vi "PFD_Heading.vi"(8 "Refresh Rate (Hz)":u32=30) -> ()   [LabVIEW 2023]
uses:
  <vilib>/Utility/miscctls.llb/LVBoundsTypeDef.ctl
  pfd_global.vi
panel:
  out "HDG":bool
  out "PFD_HeadingControl":sgl format="%#_13g"
  out "PFD_HeadingTop":picture
  out "PFD_Heading":picture
  out "PFD_HeadingBack":picture
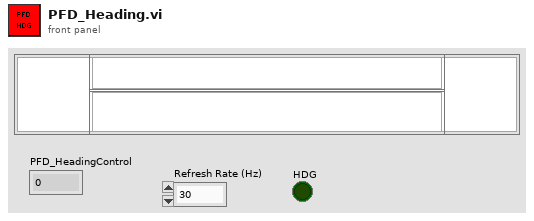
[diagram p1: front panel]
types:
  T1 = cluster{"left":i16, "top":i16, "right":i16, "bottom":i16}
  T2 = typedef "LVBoundsTypeDef.ctl" = cluster{"Width":u32, "Height":u32}
  T3 = cluster{"Font Name:":string, "Size":i16, "Strikeout?":bool, "Italic?":bool, "Underline?":bool, "Outline?":bool, "Shadow?":bool, "Bold?":bool}
  T4 = enum16{"User-specified Font", "Application Font", "System Font", "Dialog Font"}
  T5 = cluster{"horizontal":enum16{"left", "center", "right"}, "vertical":enum16{"top", "center", "bottom"}}
  T6 = cluster{cluster{i16, "x":i16}, cluster{i16, "x":i16}}
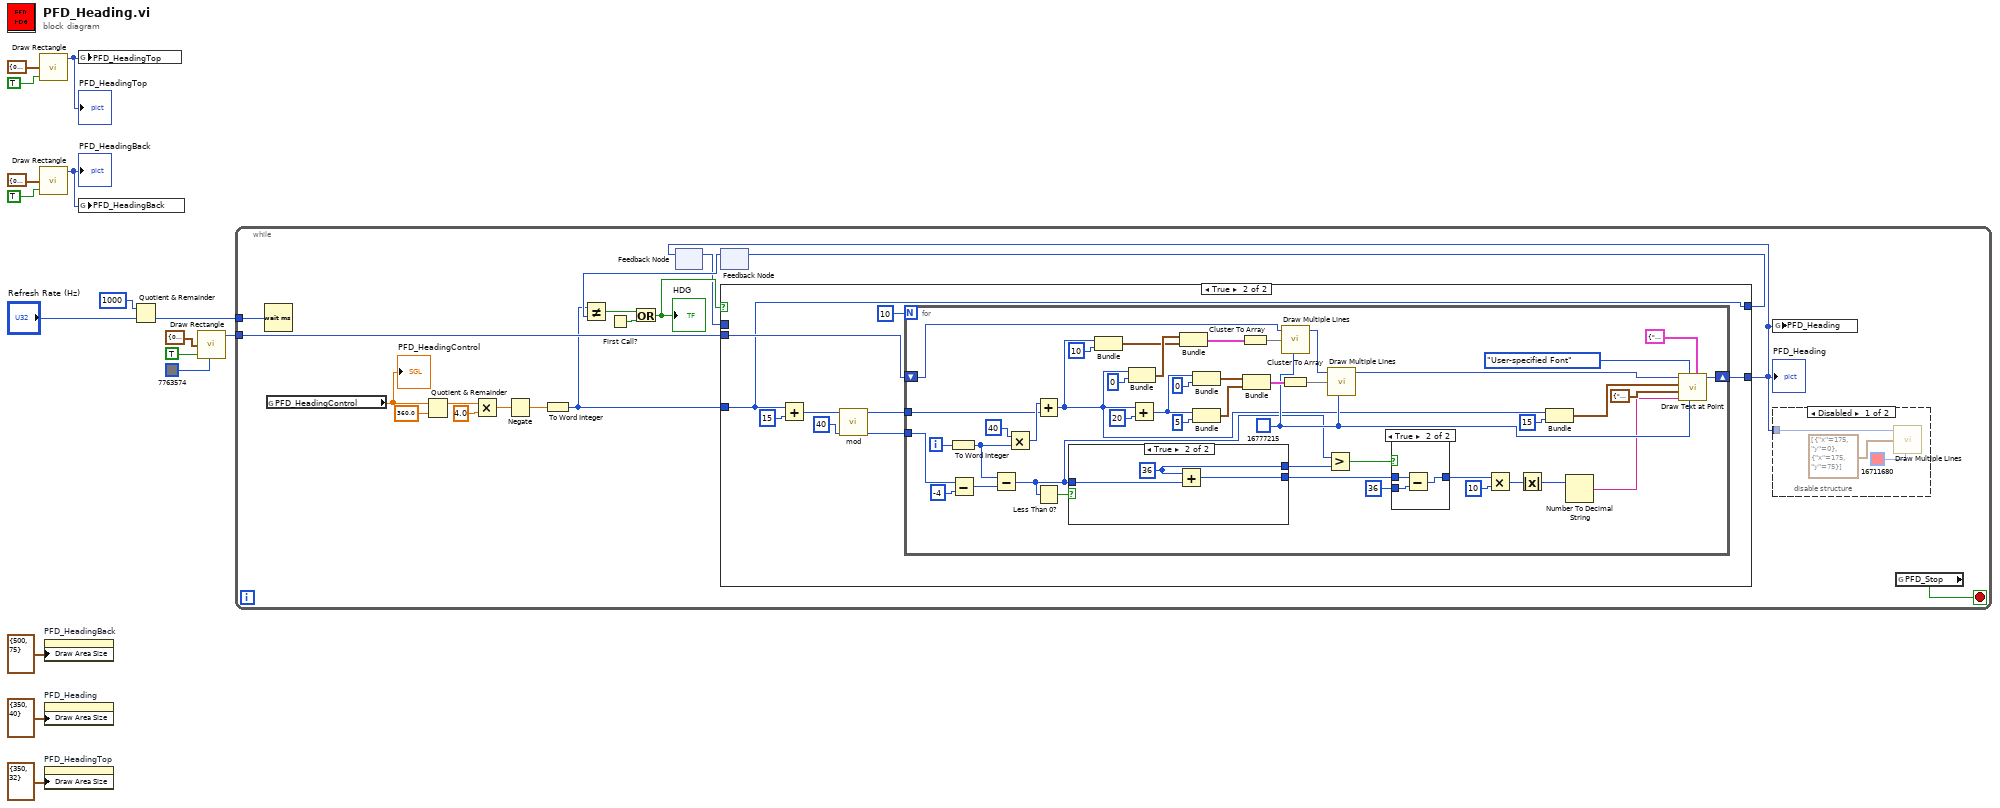
[diagram p0: block diagram]
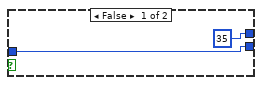
[diagram p5: hidden frame]
diagram:
  n1 = call <vilib>:"Draw Rectangle.vi"("rect"=T1 {"left"=0, "top"=0, "right"=350, "bottom"=52}, "fill?(F)"=TRUE) -> ("new picture"=w2:picture)  [unwired: 7 in]
  "PFD_HeadingTop" <- w2
  n2 = call <vilib>:"Draw Rectangle.vi"("rect"=T1 {"left"=0, "top"=0, "right"=500, "bottom"=75}, "fill?(F)"=TRUE) -> ("new picture"=w1:picture)  [unwired: 7 in]
  "PFD_HeadingBack" <- w1
  n3 = property on="PFD_HeadingBack" class="Pict"("Draw Area Size"=T2 {"Width"=500, "Height"=75}) -> ()  [unwired: 2 in, 2 out]
  n4 = property on="PFD_Heading" class="Pict"("Draw Area Size"=T2 {"Width"=350, "Height"=40}) -> ()  [unwired: 2 in, 2 out]
  n5 = property on="PFD_HeadingTop" class="Pict"("Draw Area Size"=T2 {"Width"=350, "Height"=32} ("Draw Area Size 2")) -> ()  [unwired: 2 in, 2 out]
  n6 = global write "PFD_global.vi" "PFD_HeadingTop"(w2) -> ()
  n7 = global write "PFD_global.vi" "PFD_HeadingBack"(w1) -> ()
  n8 = Quotient & Remainder(x=u32 1000, y="Refresh Rate (Hz)") -> (floor(x/y)=w3:u32)  [unwired: 1 out]
  n9 = call <vilib>:"Draw Rectangle.vi"("rect"=T1 {"left"=0, "top"=0, "right"=350, "bottom"=40}, "fill?(F)"=TRUE, "color(black)"=u32 7763574 ("color_Background")) -> ("new picture"=w10:picture)  [unwired: 6 in]
  n10 = while {
    tunnel: w10 -> [w33]
    tunnel: w3 -> [w20]
    stop <- w17 stop-if-true
    n11 = Wait (ms)(milliseconds to wait=w20) -> ()  [unwired: 1 out]
    n12 = global read "PFD_global.vi" "PFD_HeadingControl"() -> (w19:sgl)
    "PFD_HeadingControl" <- w19
    n13 = Quotient & Remainder(x=w19, y=sgl 360.0) -> (x-y*floor(x/y)=w25:sgl)  [unwired: 1 out]
    n14 = Multiply(x=w25, y=sgl 4.0) -> (x*y=w24:sgl)
    n15 = Negate(x=w24) -> (-x=w26:sgl)
    n16 = To Word Integer(number=w26) -> (16bit integer=w21:i16)
    n17 = First Call?() -> (First Call?: T/F=w31:bool)
    n18 = feedback #1() -> (w27:picture)  [unwired: 1 in]
    n19 = feedback #2() -> (w28:i16)  [unwired: 1 in]
    n20 = Not Equal?(x=w21, y=w28) -> (x != y?=w32:bool)
    n21 = Or(x=w32, y=w31) -> (x .or. y?=w30:bool)
    "HDG" <- w30
    n22 = case shown="True" w30 {
      tunnel: [w38 w46] -> w18
      tunnel: w33 -> [_ w45]
      tunnel: [w37 w39] -> w29
      tunnel: w27 -> [w38 _]
      tunnel: w21 -> [w37 w39]
      frame False {
      }
      frame True {
        n23 = Add(x=w39, y=i16 15) -> (x+y=w44:i16)
        n24 = call "mod.vi"("Divide"=i16 40 ("x"), "Value In"=w44) -> ("Ceil"=w41:i16, "Value out"=w40:i16)  [unwired: 8 in]
        n25 = for {
          N: 10 ("Numeric") -> [_]
          shift-right: [w76] -> w46
          shift-left: w45 -> [w91]
          tunnel: w41 -> [w51]
          tunnel: w40 -> [w50]
          i -> [w89]
          w75 = u32 16777215 ("color(black)")
          n26 = To Word Integer(number=w89) -> (16bit integer=w71:i16)
          n27 = Subtract(x=w51, y=i16 -4) -> (x-y=w64:i16)
          n28 = Subtract(x=w71, y=w64) -> (x-y=w57:i16)
          n29 = Multiply(x=i16 40, y=w71) -> (x*y=w72:i16)
          n30 = Add(x=w72, y=w50) -> (x+y=w74:i16)
          n31 = Less Than 0?(x=w57) -> (x < 0?=w58:bool)
          n32 = case shown="True" w58 {
            tunnel: w57 -> [w97 w99]
            tunnel: [w97 w100] -> w60
            tunnel: [i16 35 ("y") w98] -> w48
            frame False {
            }
            frame True {
              w98 = i16 36 ("y")
              n33 = Add(x=w98, y=w99) -> (x+y=w100:i16)
            }
          }
          n34 = Bundle(w74, "x"=i16 10) -> (w86:cluster{i16, "x":i16})  [unwired: 1 in]
          n35 = Bundle(w74, "x"=i16 0) -> (w87:cluster{i16, "x":i16})  [unwired: 1 in]
          n36 = Add(x=w74, y=i16 20) -> (x+y=w78:i16)
          n37 = Bundle(w87, w86) -> (w85:T6)  [unwired: 1 in]
          n38 = Bundle(w78, "x"=i16 0) -> (w79:cluster{i16, "x":i16})  [unwired: 1 in]
          n39 = Bundle(w78, "x"=i16 5) -> (w81:cluster{i16, "x":i16})  [unwired: 1 in]
          n40 = Cluster To Array(cluster=w85) -> (array=w84:cluster{i16, "x":i16}[])
          n41 = Bundle(w79, w81) -> (w80:T6)  [unwired: 1 in]
          n42 = Cluster To Array(cluster=w80) -> (array=w69:cluster{i16, "x":i16}[])
          n43 = call <vilib>:"Draw Multiple Lines.vi"("picture"=w91, "line endpoints"=w84, "color(black)"=w75) -> ("new picture"=w70:picture)  [unwired: 6 in]
          n44 = Greater?(x=w57, y=w48) -> (0:w59:bool)
          n45 = call <vilib>:"Draw Multiple Lines.vi"("picture"=w70, "line endpoints"=w69, "color(black)"=w75) -> ("new picture"=w68:picture)  [unwired: 6 in]
          n46 = case shown="True" w59 {
            tunnel: i16 36 ("y") -> [_ w95]
            tunnel: w60 -> [w92 w94]
            tunnel: [w92 w93] -> w54
            frame False {
            }
            frame True {
              n47 = Subtract(x=w94, y=w95) -> (x-y=w93:i16)
            }
          }
          n48 = Multiply(x=w54, y=i16 10) -> (x*y=w52:i16)
          n49 = Absolute Value(x=w52) -> (abs(x)=w56:i16)
          n50 = Bundle(w74, "x"=i16 15) -> (w66:cluster{i16, "x":i16})  [unwired: 1 in]
          n51 = Number To Decimal String(number=w56) -> (decimal integer string=w55:string)  [unwired: 1 in]
          n52 = call <vilib>:"Draw Text at Point.vi"("[user-specified font]"=T3 {"Font Name:"="a", "Size"=18, "Strikeout?"=FALSE, "Italic?"=FALSE, "Underline?"=FALSE, "Outline?"=FALSE, "Shadow?"=FALSE, "Bold?"=TRUE}, "text color(black)"=w75, "desired font(Application)"=T4."User-specified Font", "text"=w55, "alignment(left, top)"=T5 {"horizontal"=enum."center", "vertical"=enum."top"}, "origin"=w66, "picture"=w68) -> ("new picture"=w76:picture)  [unwired: 3 in, 1 out]
        }
      }
    }
    "PFD_Heading" <- w18
    n53 = feedback-in #1(w18) -> ()
    n54 = feedback-in #2(w29) -> ()
    n55 = global write "PFD_global.vi" "PFD_Heading"(w18) -> ()
    n56 = disable-structure shown="Disabled" {
      disable-tunnel: w18 -> [w34 _]
      frame Disabled {
        n57 = call <vilib>:"Draw Multiple Lines.vi"("picture"=w34, "line endpoints"=cluster{"x":i16, "y":i16}[] [{"x"=175, "y"=0}, {"x"=175, "y"=75}], "color(black)"=u32 16711680) -> ()  [unwired: 6 in, 1 out]
      }
      frame Enabled {
      }
    }
    n58 = global read "PFD_global.vi" "PFD_Stop"() -> (w17:bool)
  }
